vi "Drive Modifications.vi"(1 "Drive Global Data In":T1) -> (0 "Drive Global Data Out":T1)   [LabVIEW 2013]
panel:
  in  "Wheel Diameter(in)":dbl format="%#_13g"
  out "Revolutions right":dbl
  out "Right Distance (meter)":dbl
  out "Current right angle (deg)":dbl(knob) scale=0.0..360.0
  out "Current left angle (deg)":dbl(knob) scale=0.0..360.0
  out "left Distance (meter)":dbl
  out "Revolutions left":dbl
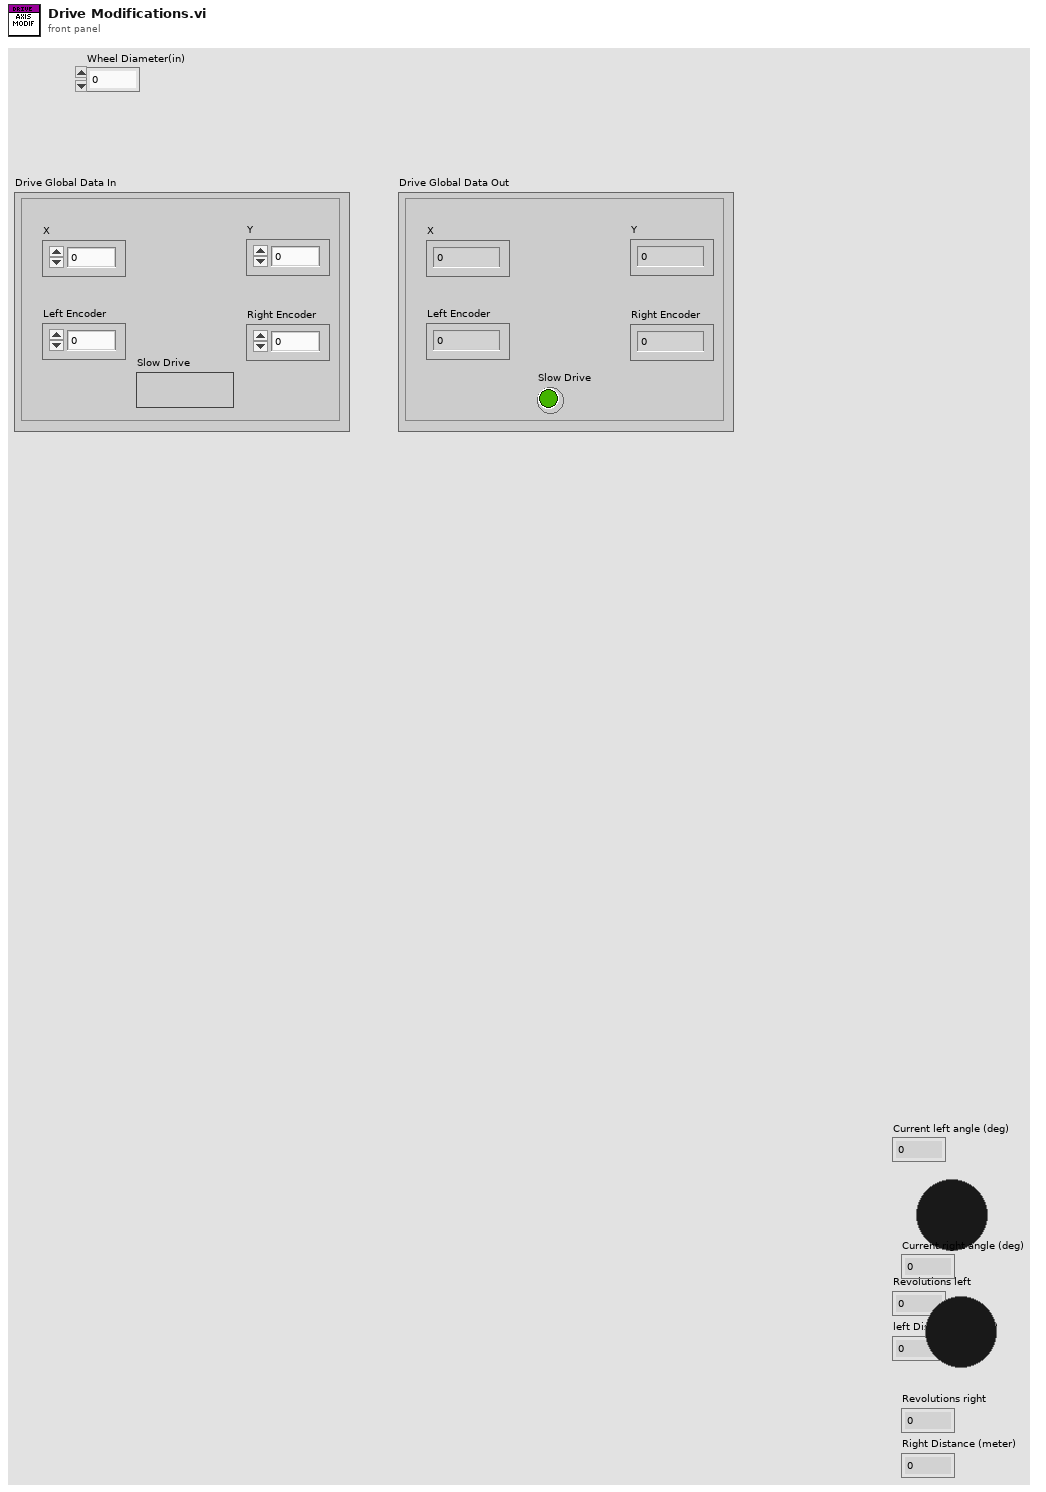
[diagram p1: front panel]
types:
  T1 = cluster{"Y":dbl, "X":dbl, "Left Encoder":dbl, "Right Encoder":dbl, "Slow Drive":bool}
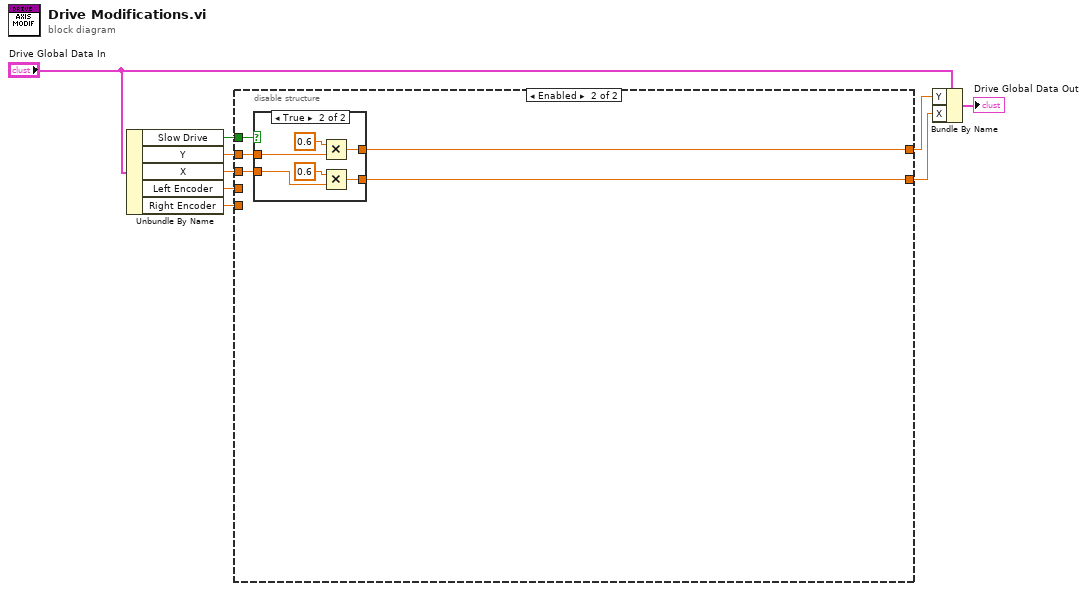
[diagram p0: block diagram]
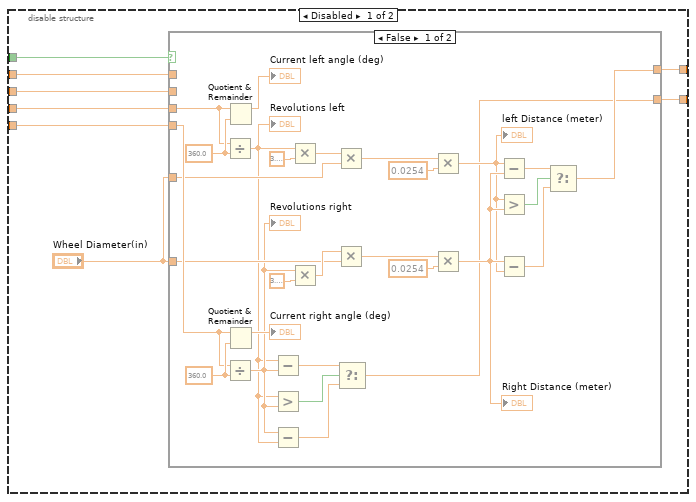
[diagram p2: hidden frame]
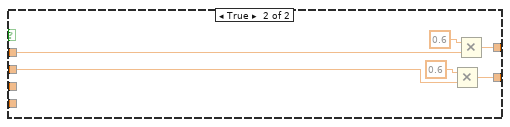
[diagram p3: hidden frame]
diagram:
  n1 = Unbundle By Name("Drive Global Data In") -> ("Slow Drive"=w5:bool, "Y"=w2:dbl, "X"=w1:dbl, "Left Encoder"=w4:dbl, "Right Encoder"=w3:dbl)
  n2 = disable-structure shown="Enabled" {
    disable-tunnel: w2 -> [w17 w53]
    disable-tunnel: w1 -> [w16 w52]
    disable-tunnel: [w15 w56] -> w7
    disable-tunnel: [w14 w55] -> w6
    disable-tunnel: w5 -> [w13 w54]
    disable-tunnel: w4 -> [w12 _]
    disable-tunnel: w3 -> [w11 _]
    frame Disabled {
      n3 = case shown="False" w13 {
        tunnel: w17 -> [_ w49]
        tunnel: w16 -> [_ w48]
        tunnel: [w24 w47] -> w15
        tunnel: [w18 w46] -> w14
        tunnel: w12 -> [w41 _]
        tunnel: w11 -> [w36 _]
        tunnel: "Wheel Diameter(in)" -> [w35 _]
        tunnel: "Wheel Diameter(in)" -> [w34 _]
        frame False {
          w37 = 360.0 ("y")
          w45 = 360.0 ("y")
          n4 = Divide(x=w41, y=w45) -> (x/y=w19:dbl)
          "Revolutions left" <- w19
          n5 = Divide(x=w36, y=w37) -> (x/y=w20:dbl)
          "Revolutions right" <- w20
          n6 = Quotient & Remainder(x=w41, y=w45) -> (x-y*floor(x/y)=→"Current left angle (deg)":dbl)  [unwired: 1 out]
          n7 = Quotient & Remainder(x=w36, y=w37) -> (x-y*floor(x/y)=→"Current right angle (deg)":dbl)  [unwired: 1 out]
          n8 = Subtract(x=w19, y=w20) -> (x-y=w22:dbl)
          n9 = Greater?(x=w19, y=w20) -> (0:w21:bool)
          n10 = Subtract(x=w20, y=w19) -> (x-y=w23:dbl)
          n11 = Multiply(x=w19, y=3.141592653589793) -> (x*y=w43:dbl)
          n12 = Multiply(x=w20, y=3.141592653589793) -> (x*y=w39:dbl)
          n13 = Multiply(x=w43, y=w35) -> (x*y=w33:dbl)
          n14 = Multiply(x=w39, y=w34) -> (x*y=w30:dbl)
          n15 = Select(t=w22, s=w21, f=w23) -> (s? t:f=w18:dbl)
          n16 = Multiply(x=w33, y=0.0254) -> (x*y=w26:dbl)
          "left Distance (meter)" <- w26
          n17 = Multiply(x=w30, y=0.0254) -> (x*y=w27:dbl)
          "Right Distance (meter)" <- w27
          n18 = Subtract(x=w26, y=w27) -> (x-y=w28:dbl)
          n19 = Greater?(x=w26, y=w27) -> (0:w29:bool)
          n20 = Subtract(x=w27, y=w26) -> (x-y=w25:dbl)
          n21 = Select(t=w28, s=w29, f=w25) -> (s? t:f=w24:dbl)
        }
        frame True {
          n22 = Multiply(x=0.6 ("t"), y=w48) -> (x*y=w46:dbl)
          n23 = Multiply(x=0.6 ("t"), y=w49) -> (x*y=w47:dbl)
        }
      }
    }
    frame Enabled {
      n24 = case shown="True" w54 {
        tunnel: w53 -> [w58 w62]
        tunnel: w52 -> [w57 w59]
        tunnel: [w58 w61] -> w56
        tunnel: [w57 w60] -> w55
        frame False {
        }
        frame True {
          n25 = Multiply(x=0.6 ("t"), y=w62) -> (x*y=w61:dbl)
          n26 = Multiply(x=0.6 ("t"), y=w59) -> (x*y=w60:dbl)
        }
      }
    }
  }
  n27 = Bundle By Name(cluster="Drive Global Data In", "Y"=w7, "X"=w6) -> (→"Drive Global Data Out":T1)
